vi "Lecture_Fichiers.vi"() -> ()   [LabVIEW 2018]
panel:
  out "spreadsheet string":string
  out "String":string
  out "sorted array":string[](array[string])
  out "array":string[](array[string])
  out "appended path":path
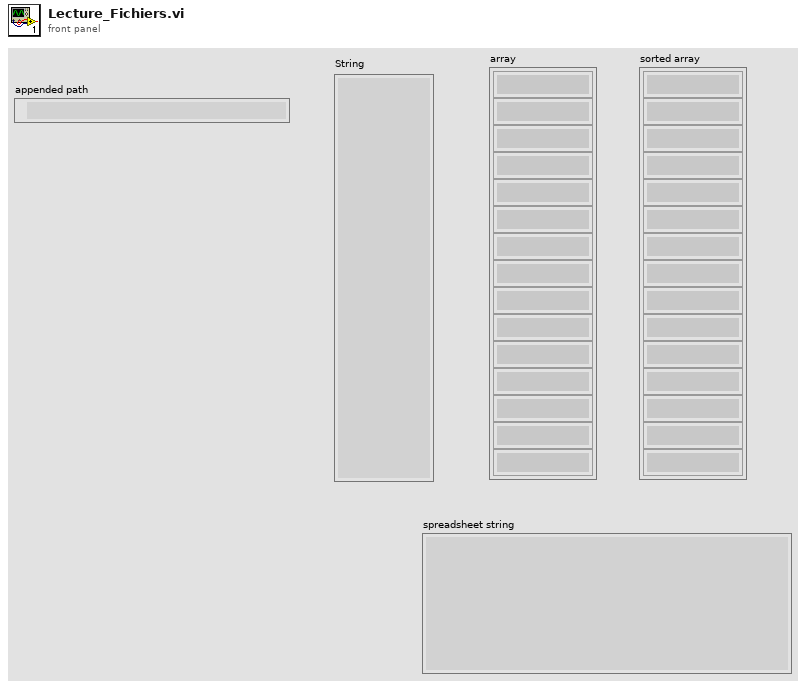
[diagram p1: front panel]
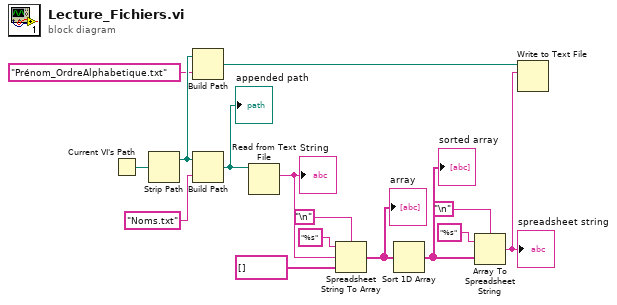
[diagram p0: block diagram]
diagram:
  n1 = Current VI's Path() -> (path=w15:path)
  n2 = Strip Path(path=w15) -> (stripped path=w3:path)  [unwired: 1 out]
  n3 = Build Path(base path=w3, name or relative path="Prénom_OrdreAlphabetique.txt") -> (appended path=w1:path)
  n4 = Build Path(base path=w3, name or relative path="Noms.txt") -> (appended path=w13:path)
  "appended path" <- w13
  n5 = Read from Text File(file (use dialog)=w13) -> (text=w8:string)  [unwired: 3 in, 3 out]
  "String" <- w8
  n6 = Spreadsheet String To Array(delimiter (Tab)="\n", format string="%s", spreadsheet string=w8, array type (2D Dbl)=string[] []) -> (array=w9:string[])
  "array" <- w9
  n7 = Sort 1D Array(array=w9) -> (sorted array=w7:string[])
  "sorted array" <- w7
  n8 = Array To Spreadsheet String(delimiter (Tab)="\n", array=w7, 3:"%s" ("format string")) -> (spreadsheet string=w4:string)
  "spreadsheet string" <- w4
  n9 = Write to Text File(file (use dialog)=w1, text=w4) -> ()  [unwired: 2 in, 3 out]
